vi "Get PPL Info.vi"(8 "Error In":errorcluster) -> (0 "Error Out":errorcluster, 1 "Build Version":string, 2 "PPL Filename":string, 3 "PPL Original Filename":string)   [LabVIEW 2023, in "PowerModuleInterface.lvlib" / "PowerModuleInterface.lvclass"]
uses:
  PowerModuleInterface.lvclass
  <vilib>/Utility/LVLibp/NI_PackedLibraryUtility.lvlib
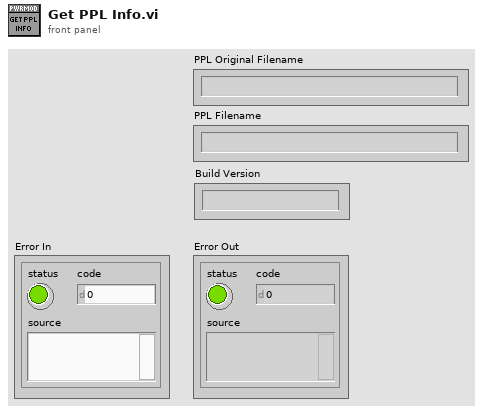
[diagram p1: front panel]
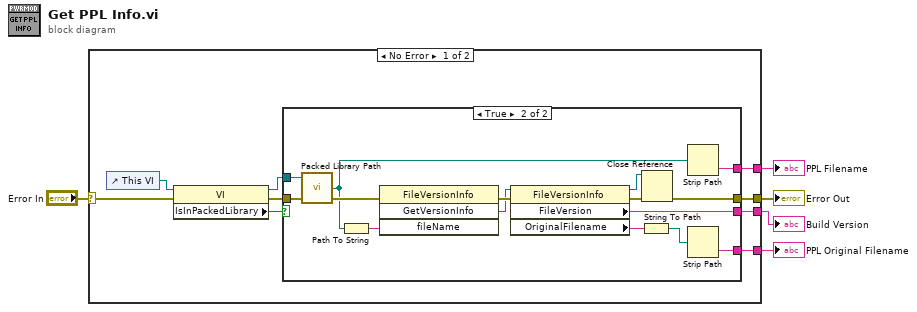
[diagram p0: block diagram]
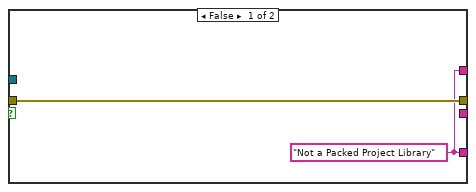
[diagram p2: hidden frame]
diagram:
  n1 = case shown="No Error" "Error In" {
    selector: "Error In" -> [w9 w32]
    tunnel: [w10 _] -> w5
    tunnel: [w8 w32] -> w3
    tunnel: [w7 _] -> w2
    tunnel: [w6 _] -> w1
    frame No Error {
      n2 = control-ref of="This VI"() -> (w14:refnum<vi>)
      n3 = property class="VI"(reference=w14, error in=w9) -> (reference out=w12:refnum<vi>, error out=w11:errorcluster, "IsInPackedLibrary"=w13:bool)
      n4 = case shown="True" w13 {
        tunnel: w12 -> [_ w31]
        tunnel: w11 -> [w16 w30]
        tunnel: [_ w26] -> w10
        tunnel: [w16 w22] -> w8
        tunnel: [w15 w20] -> w7
        tunnel: [w15 w19] -> w6
        frame False {
          w15 = "Not a Packed Project Library" ("name")
        }
        frame True {
          n5 = call <vilib>:"Packed Library Path.vi"("error in (no error)"=w30, "vi reference"=w31) -> ("error out"=w28:errorcluster, "packed library path"=w21:path)  [unwired: 1 in, 1 out]
          n6 = Path To String(path=w21) -> (string=w29:string)
          n7 = invoke class="FileVersionInfo" method="GetVersionInfo"(error in=w28, "fileName"=w29) -> (error out=w27:errorcluster, "GetVersionInfo"=w25:refnum<k24>)  [unwired: 2 in, 2 out]
          n8 = property class="FileVersionInfo"(reference=w25, error in=w27) -> (reference out=w24:refnum<k24>, error out=w23:errorcluster, "FileVersion"=w26:string, "OriginalFilename"=w18:string)
          n9 = String To Path(string=w18) -> (path=w17:path)
          n10 = Close Reference(reference=w24, error in (no error)=w23) -> (error out=w22:errorcluster)
          n11 = Strip Path(path=w21) -> (name=w20:string)  [unwired: 1 out]
          n12 = Strip Path(path=w17) -> (name=w19:string)  [unwired: 1 out]
        }
      }
    }
    frame Error {
    }
  }
  "Build Version" <- w5
  "Error Out" <- w3
  "PPL Filename" <- w2
  "PPL Original Filename" <- w1
